vi "init_parameters.vi"() -> (1 "Numeric":i32, 2 "remote port or service name":u16, 3 "String":string)   [LabVIEW 2018, in "ESP301_via_TCPIP.lvclass"]
uses:
  ESP301_via_TCPIP.lvclass
panel:
  in  "OK Button":bool
  in  "Numeric 2":i32=10000
  in  "remote port or service name 2":u16=5002
  in  "String 2":string="10.152.212.240"
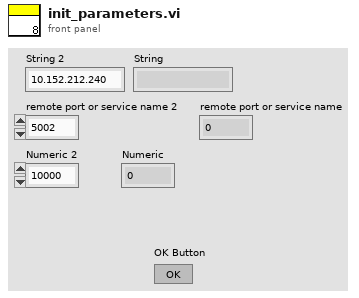
[diagram p1: front panel]
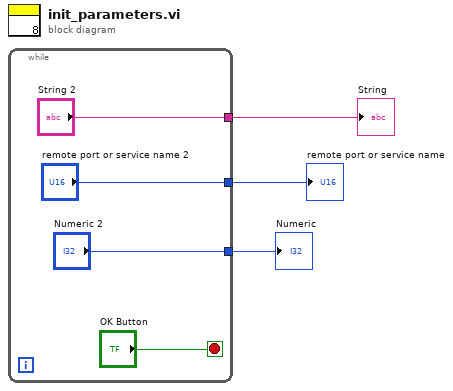
[diagram p0: block diagram]
diagram:
  n1 = while {
    tunnel: ["remote port or service name 2"] -> w3
    tunnel: ["Numeric 2"] -> w2
    tunnel: ["String 2"] -> w1
    stop <- "OK Button" stop-if-true
  }
  "remote port or service name" <- w3
  "Numeric" <- w2
  "String" <- w1
